vi "Table Background Color All Parameter.vi"(9 "单元格背景色":u32(colorbox), 10 "行":i32, 11 "列":i32) -> (3 "活动单元格":cluster{cluster{i32, i32}, "单元格背景色":u32}[](array[cluster]))   [LabVIEW 2015, in "Utility VIs.lvlib"]
uses:
  Utility VIs.lvlib
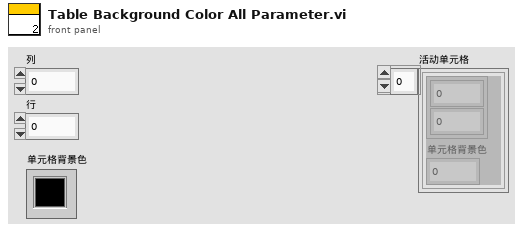
[diagram p1: front panel]
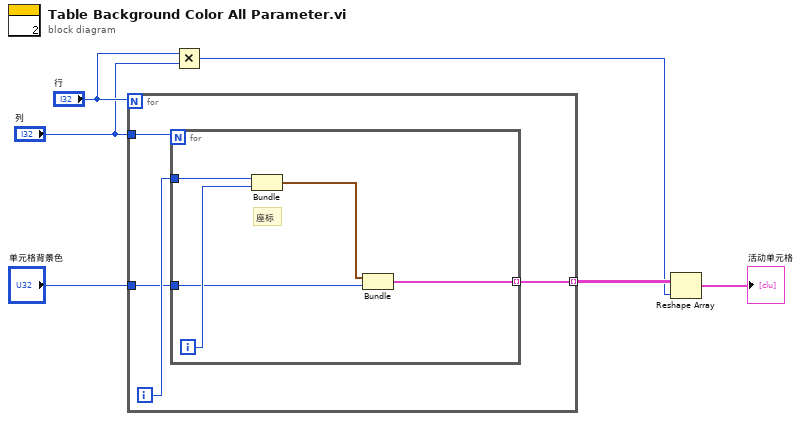
[diagram p0: block diagram]
diagram:
  n1 = for {
    N: "行" -> [_]
    tunnel: "列" -> [w10]
    tunnel: "单元格背景色" -> [w8]
    tunnel: [w7] -> w5 mode=indexing
    i -> [w9]
    n2 = for {
      N: w10 -> [_]
      tunnel: w9 -> [w15]
      tunnel: w8 -> [w12]
      tunnel: [w11] -> w7 mode=indexing
      i -> [w14]
      # "座标"
      n3 = Bundle(w15, w14) -> (w13:cluster{i32, i32})  [unwired: 1 in]
      n4 = Bundle(w13, "单元格背景色"=w12) -> (w11:cluster{cluster{i32, i32}, "单元格背景色":u32})  [unwired: 1 in]
    }
  }
  n5 = Multiply(x="行", y="列") -> (x*y=w2:i32)
  n6 = Reshape Array(w5, w2) -> (→"活动单元格":cluster{cluster{i32, i32}, "单元格背景色":u32}[])
